vi "FitParabola3 (SubVI).vi"(0 "x values":dbl[](array[numeric])=[13.399933, 13.44983225, 13.5001315, 13.55013075, 13.59993, 13.65002925, 13.7001285, 13.75002775, 13.800127, 13.84992625, 13.9000255, 13.95002475, 13.999924, 14.0500207, 14.1000174, 14.1499141, 14.2001108, 14.2500075, 14.2998042, 14.3501009, 14.3999976, 14.4497943, 14.499991, 14.5498877, 14.6000844, 14.6499811, 14.6997778, 14.7500745, 14.8000712, 14.8498679, 14.8999646, 14.9500613, 14.999958, 15.0501404, 15.1001228, 15.1501052, 15.2002876, 15.25017, 15.3001524, 15.3502348, 15.4000172, 15.4501996, 15.500082, 15.5498644, 15.6002468, 15.6502292, 15.6999116, 15.750094, 15.8001764, 15.8498588, 15.9001412, 15.9500236, 15.999906, 16.05021475, 16.0999235, 16.15003225, 16.200241, 16.25004975, 16.3000585, 16.34996725, 16.399876, 16.45018475, 16.5001935, 16.54990225], 1 "y values":dbl[](array[numeric])=[42.648277282714844, 43.9074821472168, 44.95804977416992, 46.04310607910156, 46.7999382019043, 47.876556396484375, 48.90898513793945, 49.69123077392578, 50.29452896118164, 50.99095153808594, 51.3321533203125, 52.05470657348633, 52.37543869018555, 52.83419418334961, 53.5294303894043, 53.09951400756836, 52.98366928100586, 52.9737663269043, 52.82147216796875, 52.25721740722656, 51.93815612792969, 50.699134826660156, 50.42073440551758, 49.25381088256836, 48.3885383605957, 47.47373580932617, 46.43144226074219, 45.583709716796875, 43.905120849609375, 42.53858184814453, 41.602542877197266, 40.06209182739258, 39.04403305053711, 37.436161041259766, 36.6154899597168, 35.539791107177734, 34.32120132446289, 33.28242874145508, 32.38603210449219, 31.3276309967041, 30.748254776000977, 29.91518783569336, 29.445737838745117, 28.354888916015625, 28.009984970092773, 27.285934448242188, 27.04413414001465, 26.576818466186523, 25.898874282836914, 25.55618667602539, 25.26278305053711, 24.908693313598633, 25.03961753845215, 24.513620376586914, 24.64219093322754, 25.168533325195312, 24.8322811126709, 25.24604606628418, 25.068620681762695, 25.58075714111328, 25.197729110717773, 25.184911727905273, 25.455291748046875, 25.335906982421875], 2 "delta y values":dbl[](array[numeric])=[1.0, 1.0, 1.0, 1.0, 1.0, 1.0, 1.0, 1.0, 1.0, 1.0, 1.0, 1.0, 1.0, 1.0, 1.0, 1.0, 1.0, 1.0, 1.0, 1.0, 1.0, 1.0, 1.0, 1.0, 1.0, 1.0, 1.0, 1.0, 1.0, 1.0, 1.0, 1.0, 1.0, 1.0, 1.0, 1.0, 1.0, 1.0, 1.0, 1.0, 1.0, 1.0, 1.0, 1.0, 1.0, 1.0, 1.0, 1.0, 1.0, 1.0, 1.0, 1.0, 1.0, 1.0, 1.0, 1.0, 1.0, 1.0, 1.0, 1.0, 1.0, 1.0, 1.0, 1.0], 5 "error in":errorcluster, 6 "Fit type":T2, 7 "confidence level":dbl=0.95, 8 "Poly fit algorithm":T4 items=["SVD", "Givens", "Givens2", "Householder", "LU Decomposition", "Cholesky", "SVD for Rank Deficient H"], 10 "Polynomial Coefficient Constraint":cluster{"order":i32, "coefficient":dbl}[](array[cluster]), 12 "Minimization inputs":T5={"Minimizing alg"=0, "Search accuracy"=1e-08, "Step type"=0} {"Step type" items=["fixed function", "modified function"]; "Search accuracy" format="%.2e"; "Minimizing alg" items=["Golden Section Search", "Brent with Derivatives"]}) -> (14 "Plot":T6, 15 "Optimized position":dbl, 16 "Uncertainty on position":dbl, 19 "error out":errorcluster)   [LabVIEW 2016]
uses:
  Utils/Controls/Graph_TypeDef_XY.ctl
  <vilib>/Analysis/6fits.llb/General Linear Fit Algorithm.ctl
  <vilib>/Analysis/6fits.llb/Curve Fitting Criteria.ctl
  Utils/Controls/All_Enums/Enum_TypeDef_ParabolaFitType.ctl
  <vilib>/Analysis/6fits.llb/Confidence Interval (Polynomial).vi
  <vilib>/Analysis/NI_AALPro.lvlib
  <vilib>/gmath/NI_Gmath.lvlib
panel:
  out "Y error bars":cluster{dbl[], dbl[]}(graph)
  in  "Tab Control":T1(tab)
  in  "Quadratic fit method":T3 items=["Least Square", "Least Absolute Residual", "Bisquare"]
  out "Delta Polynomial Coefficients":dbl[](array[numeric])
  out "Fitted quadratic":string
  out "f(optimized position)":dbl[](array[numeric]) format="%.2f"
  out "Best Quadratic Fit":dbl[](array[numeric])
  out "Poly fit residue":dbl
  out "Polynomial Coefficients":dbl[](array[numeric])
  # "FIT PARABOLA 3 Brandeis University - Brookhaven National Laboratory * ATLAS Phase II Inner Tracker Upgrade"
  # "-(formula) if looking for a maxium instead"
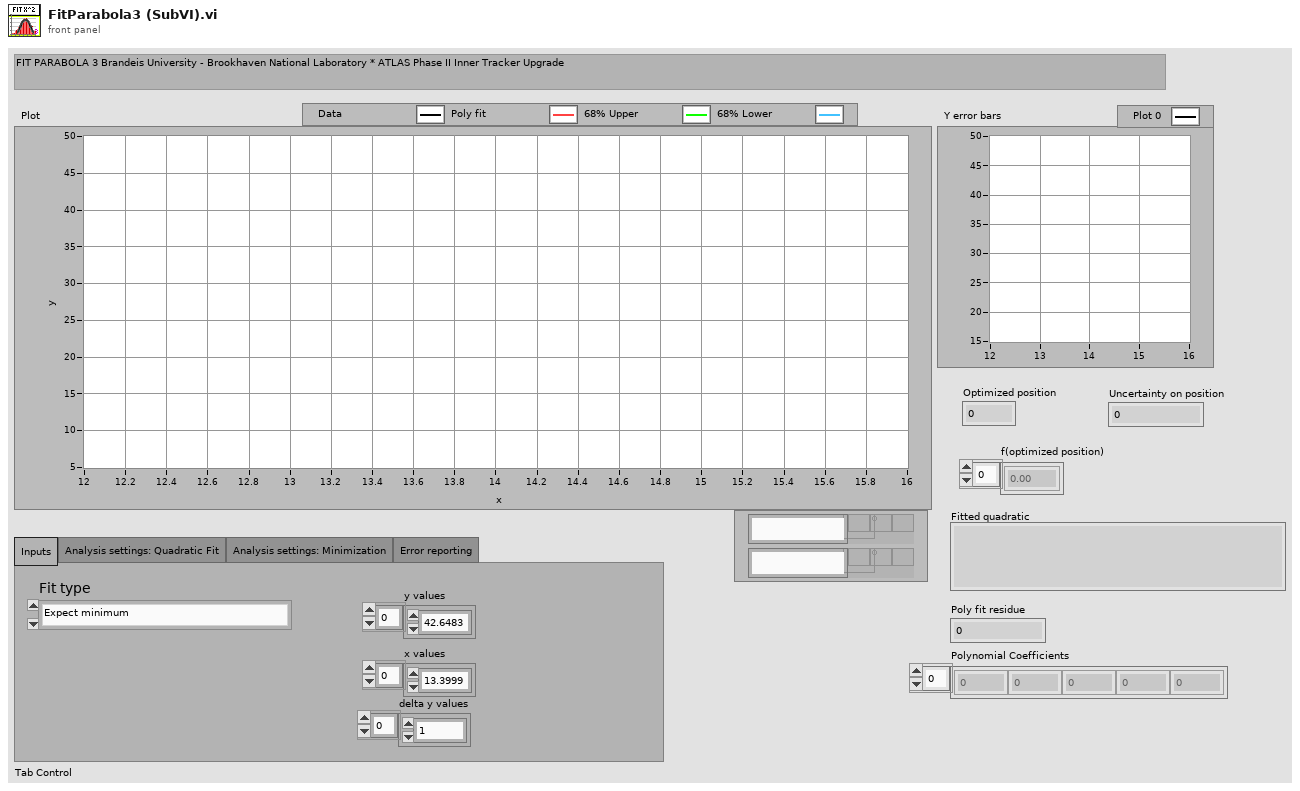
[diagram p1: front panel]
types:
  T1 = enum32{"Inputs", "Analysis settings: Quadratic Fit", "Analysis settings: Minimization", "Error reporting"}
  T2 = typedef "Enum_TypeDef_ParabolaFitType.ctl" = enum16{"Expect minimum", "Expect maximum"}
  T3 = typedef "NI_AALPro.lvlib/Curve Fitting Criteria.ctl" = u16
  T4 = typedef "NI_AALPro.lvlib/General Linear Fit Algorithm.ctl" = u16
  T5 = cluster{"Minimizing alg":u16, "Search accuracy":dbl, "Step type":u16}
  T6 = typedef "Graph_TypeDef_XY.ctl" = cluster{"Radius bins":dbl[], "Best Gaussian Fit":dbl[]}[]
  T7 = typedef "Enum_TypeDef_Tails.ctl" = enum16{"No tails", "Left tail", "Right tail"}
  T8 = cluster{"Selected x values":dbl[], "Best Quadratic Fit":dbl[]}
  T9 = cluster{"Selected x values":dbl[], "Upper Bound":dbl[]}
  T10 = cluster{"Selected x values":dbl[], "Lower Bound":dbl[]}
  T11 = cluster{"Selected x values":dbl[], "Lower Bound":dbl[]}[]
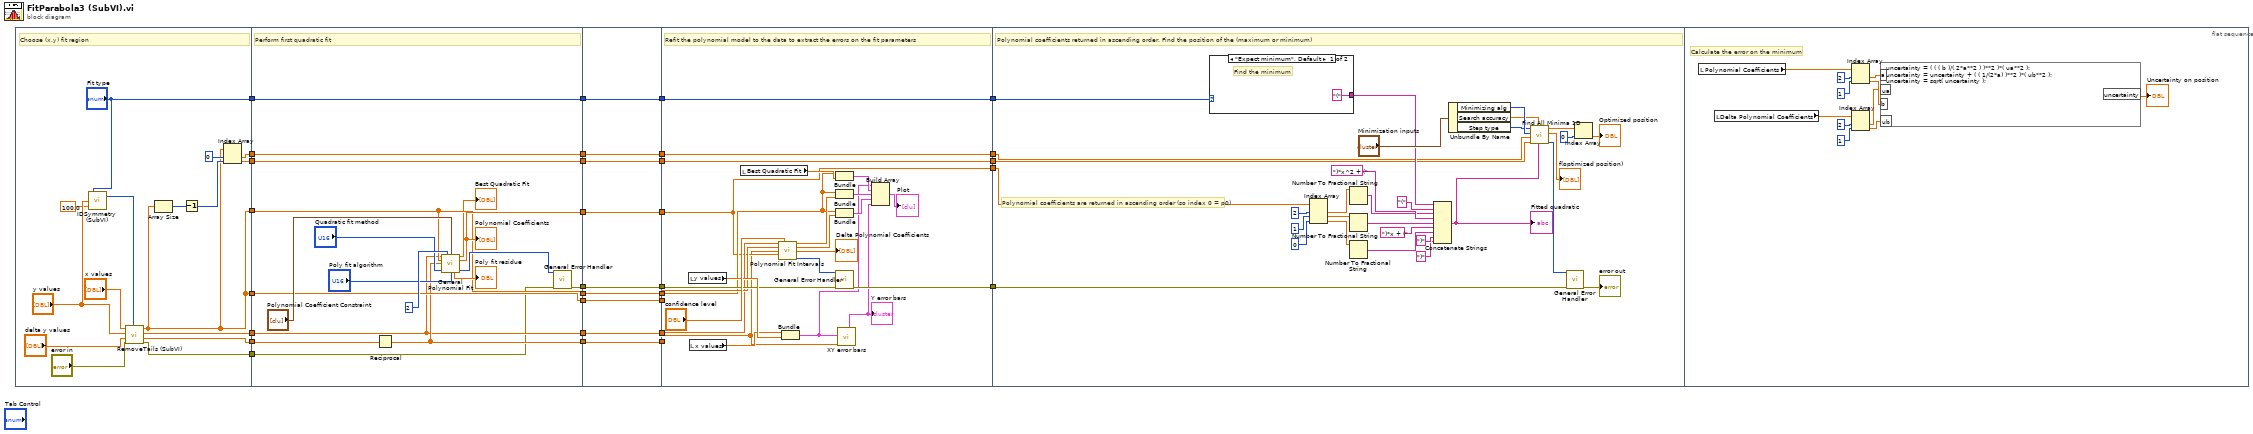
[diagram p0: block diagram]
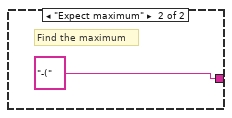
[diagram p2: hidden frame]
diagram:
  n1 = flat-sequence {
    tunnel: [w40] -> w30
    tunnel: [w38] -> w29
    tunnel: [w39] -> w28
    tunnel: [w40] -> w27
    tunnel: [w44] -> w25
    tunnel: [w43] -> w24
    tunnel: ["Fit type"] -> w21
    tunnel: [w32] -> w1
    tunnel: [w63] -> w19
    tunnel: [w59] -> w17
    tunnel: w30 -> [w56]
    tunnel: w29 -> [w57]
    tunnel: w28 -> [w49]
    tunnel: [w56] -> w15
    tunnel: [w49] -> w13
    tunnel: [w51] -> w11
    tunnel: w27 -> [w55]
    tunnel: [w55] -> w9
    tunnel: w25 -> [w54]
    tunnel: w24 -> [w53]
    tunnel: [w54] -> w7
    tunnel: [w53] -> w5
    tunnel: w21 -> [w52]
    tunnel: [w52] -> w3
    tunnel: w1 -> [w48]
    tunnel: w19 -> [w74]
    tunnel: [w74] -> w18
    tunnel: w17 -> [w73]
    tunnel: [w73] -> w16
    tunnel: w15 -> [w72]
    tunnel: [w72] -> w14
    tunnel: w13 -> [w71]
    tunnel: [w71] -> w12
    tunnel: w11 -> [w70]
    tunnel: [w70] -> w10
    tunnel: w9 -> [w69]
    tunnel: [w69] -> w8
    tunnel: w7 -> [w68]
    tunnel: [w68] -> w6
    tunnel: w5 -> [w67]
    tunnel: [w67] -> w4
    tunnel: w3 -> [w66]
    tunnel: [w66] -> w2
    tunnel: w18 -> [w89]
    tunnel: w16 -> [w80]
    tunnel: [w88] -> w31
    tunnel: w14 -> [w86]
    tunnel: w12 -> [w85]
    tunnel: w10 -> [w77]
    tunnel: w8 -> [w84]
    tunnel: [w80] -> w26
    tunnel: w6 -> [w79]
    tunnel: w4 -> [w78]
    tunnel: [w79] -> w23
    tunnel: [w78] -> w22
    tunnel: [w76] -> w20
    tunnel: w2 -> [w76]
    tunnel: w31 -> [w112]
    tunnel: w26 -> [w107]
    tunnel: w23 -> [w104]
    tunnel: w22 -> [w103]
    tunnel: w20 -> [w102]
    frame #0 {
      # "Choose (x,y) fit region"
      n2 = call "IDSymmetry (SubVI).vi"("Tolerance (%)"=100.0, "Values"="y values", "Fit type"="Fit type") -> ("Side of Tail"=w35:T7)  [unwired: 1 out]
      n3 = call "RemoveTails (SubVI).vi"("Side of Tail"=w35, "error in (no error)"="error in", "delta y values"="delta y values", "y values"="y values", "x values"="x values") -> ("error out"=w32:errorcluster, "Selected delta y values"=w38:dbl[], "Selected y values"=w39:dbl[], "Selected x values"=w40:dbl[])  [unwired: 3 in]
      n4 = Array Size(array=w40) -> (size(s)=w46:i32)
      n5 = Decrement(x=w46) -> (x-1=w47:i32)
      n6 = Index Array(array=w40, index #1=0 ("index"), index #2=w47) -> (element #1=w44:dbl, element #2=w43:dbl)
    }
    frame #1 {
      # "Perform first quadratic fit"
      n7 = Reciprocal(x=w57) -> (1/x=w51:dbl[])
      n8 = call <vilib>:"General Polynomial Fit.vi"("Y"=w49, "polynomial order"=2, "Coefficient Constraint"="Polynomial Coefficient Constraint", "X"=w56, "Weight"=w51, "method"="Quadratic fit method", "algorithm"="Poly fit algorithm") -> ("Best Polynomial Fit"=→"Best Quadratic Fit":dbl[], "Polynomial Coefficients"=w59:dbl[], "residue"=→"Poly fit residue":dbl, "error"=w64:i32)  [unwired: 5 in]
      "Polynomial Coefficients" <- w59
      n9 = call <vilib>:"General Error Handler.vi"("[error code] (0)"=w64, "error in (no error)"=w48) -> ("error out"=w63:errorcluster)  [unwired: 9 in, 4 out]
    }
    frame #2 {
    }
    frame #3 {
      # "Refit the polynomial model to the data to extract the errors on the fit parameters"
      n10 = local read "y values"() -> (w97:dbl[])
      n11 = local read "x values"() -> (w83:dbl[])
      n12 = local read "Best Quadratic Fit"() -> (w96:dbl[])
      n13 = call-poly <vilib>:"Polynomial Fit Intervals.vi"("Y"=w85, "confidence level"="confidence level", "X"=w86, "Weight"=w77, "Polynomial Coefficients"=w80) -> ("Upper Bound"=w95:dbl[], "Lower Bound"=w94:dbl[], "Delta Polynomial Coefficients"=→"Delta Polynomial Coefficients":dbl[], "error"=w90:i32)  [unwired: 7 in]
      n14 = Bundle("x values"=w83, "y values"=w97) -> (w81:cluster{"x values":dbl[], "y values":dbl[]})  [unwired: 1 in]
      n15 = Bundle("Selected x values"=w84, "Best Quadratic Fit"=w96) -> (w93:T8)  [unwired: 1 in]
      n16 = Bundle("Selected x values"=w84, "Upper Bound"=w95) -> (w92:T9)  [unwired: 1 in]
      n17 = Bundle("Selected x values"=w84, "Lower Bound"=w94) -> (w91:T10)  [unwired: 1 in]
      n18 = call <vilib>:"General Error Handler.vi"("[error code] (0)"=w90, "error in (no error)"=w89) -> ("error out"=w88:errorcluster)  [unwired: 9 in, 4 out]
      n19 = call "XY error bars.vi"("XY plot"=w81, "Yerror"=w77) -> ("Y error bars"=w75:cluster{dbl[], dbl[]})  [unwired: 6 in, 2 out]
      "Y error bars" <- w75
      n20 = Build Array(w81, w93, w92, w91, w75) -> (→"Plot":T11)
    }
    frame #4 {
      # "Polynomial coefficients are returned in ascending order (so index 0 = p0)"
      # "Polynomial coefficients returned in ascending order. Find the position of the (maximum or minimum)"
      n21 = case shown="\"Expect minimum\", Default" w102 {
        tunnel: ["(" "-("] -> w106
        frame "Expect minimum", Default {
          # "Find the minimum"
        }
        frame "Expect maximum" {
          # "Find the maximum"
        }
      }
      n22 = Index Array(array=w107, index #1=2 ("index"), index #2=1 ("index"), index #3=0 ("index")) -> (element #1=w115:dbl, element #2=w116:dbl, element #3=w117:dbl)
      n23 = Number To Fractional String(number=w115) -> (F-format string=w123:string)  [unwired: 3 in]
      n24 = Number To Fractional String(number=w116) -> (F-format string=w122:string)  [unwired: 3 in]
      n25 = Number To Fractional String(number=w117) -> (F-format string=w121:string)  [unwired: 3 in]
      n26 = Concatenate Strings(w106, "(" ("string"), w123, ")*x^2 + (" ("string"), w122, ")*x + (" ("string"), w121, ")" ("string"), ")" ("string")) -> (w128:string)
      "Fitted quadratic" <- w128
      n27 = Unbundle By Name("Minimization inputs") -> ("Minimizing alg"=w111:u16, "Search accuracy"=w110:dbl, "Step type"=w109:u16)
      n28 = call <vilib>:"Find All Minima 1D.vi"("formula"=w128, "accuracy"=w110, "end"=w103, "start"=w104, "algorithm"=w111, "step type"=w109) -> ("error"=w114:i32, "f(Minima)"=→"f(optimized position)":dbl[], "Minima"=w101:dbl[])  [unwired: 1 out]
      n29 = call <vilib>:"General Error Handler.vi"("[error code] (0)"=w114, "error in (no error)"=w112) -> ("error out"=→"error out":errorcluster)  [unwired: 9 in, 4 out]
      n30 = Index Array(array=w101, index=0) -> (element=→"Optimized position":dbl)
    }
    frame #5 {
      # "Calculate the error on the minimum"
      n31 = local read "Polynomial Coefficients"() -> (w139:dbl[])
      n32 = local read "Delta Polynomial Coefficients"() -> (w142:dbl[])
      n33 = Index Array(array=w139, index #1=2 ("index"), index #2=1 ("index")) -> (element #1=w136:dbl, element #2=w135:dbl)
      n34 = Index Array(array=w142, index #1=2 ("index"), index #2=1 ("index")) -> (element #1=w134:dbl, element #2=w133:dbl)
      n35 = formula code="uncertainty = ( ( ( b )/( 2*a**2 ) )**2 )*( ua**2 );\nuncertainty = uncertainty + ( ( 1/(2*a) )**2 )*( ub**2 ); \nuncertainty = sqrt( uncertainty );"("a"=w136, "b"=w135, "ua"=w134, "ub"=w133) -> ("uncertainty"=→"Uncertainty on position":dbl)
    }
  }
